vi "User Event.vi"() -> ()   [LabVIEW 2018]
doc: "This VI is an exercise in the LabVIEW Advanced course."
panel:
  out "이벤트 카운트":i16
  in  "정지":bool
  out "이벤트 발생!":bool
  in  "이벤트 발생":bool
  out "루프 1 정지":bool
  out "이벤트를 발생시키기 위한 프로그램적인 카운트 다운":u8(slide) scale=0.0..100.0
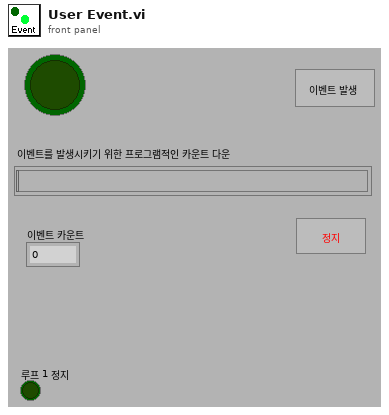
[diagram p1: front panel]
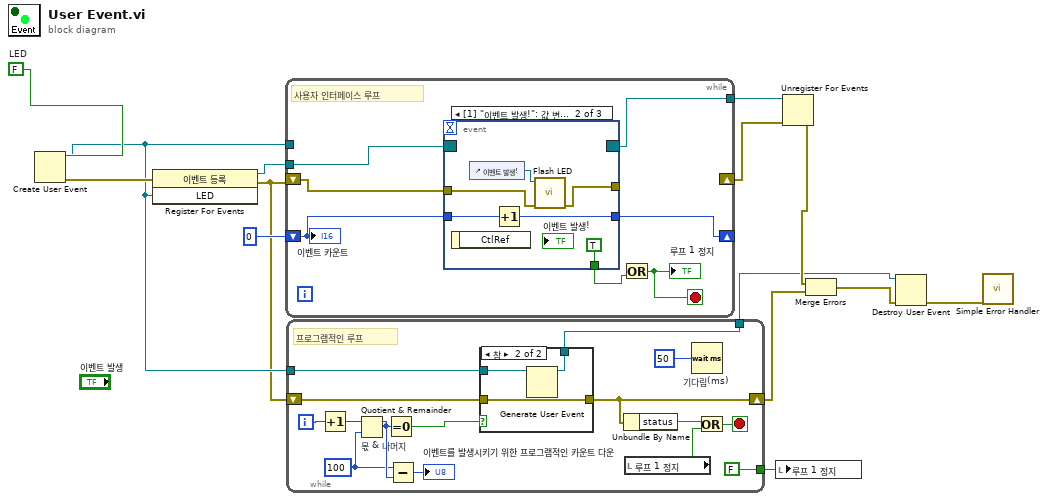
[diagram p0: block diagram]
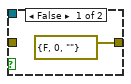
[diagram p2: hidden frame]
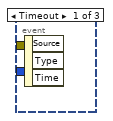
[diagram p3: hidden frame]
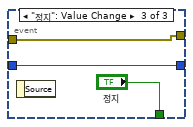
[diagram p4: hidden frame]
diagram:
  w12 = FALSE  # LED
  n1 = Create User Event(user event datatype=w12) -> (user event=w10:refnum<user-event>, error out=w11:errorcluster)  [unwired: 1 in]
  n2 = register-events(error in=w11, w10) -> (reference out=w8:refnum<event-registration>, error out=w9:errorcluster)  [unwired: 1 in]
  n3 = while {
    shift-right: [w18] -> _
    shift-left: i16 0 ("Event Count") -> [w19]
    tunnel: w10 -> [_]
    shift-right: [_] -> w7
    shift-left: w9 -> [w17]
    tunnel: w8 -> [w20]
    tunnel: [w15] -> w6
    stop <- w21 stop-if-true
    # "사용자 인터페이스 루프"
    n4 = event shown="[1] \"이벤트 발생!\": 값 변경" {
      selector: w20 -> [_ _ _]
      dyn-events: [_ _ _] -> w15
      timeout: _ -> [_ _ _]
      tunnel: w19 -> [_ w26 w29]
      tunnel: [_ w25 w29] -> w18
      tunnel: w17 -> [_ w24 w30]
      tunnel: [_ TRUE "정지"] -> w16
      tunnel: [_ w22 w30] -> _
      event Timeout {
        n5 = event-data() -> ()  [unwired: 1 in, 3 out]
      }
      event "이벤트 발생!": Value Change {
        n6 = event-data() -> ()  [unwired: 1 in, 1 out]
        n7 = control-ref of="이벤트 발생!"() -> (w27:refnum<vi>)
        n8 = Increment(x=w26) -> (x+1=w25:i16)
        n9 = call "Flash LED.vi"("에러 입력(에러 없음)"=w24, "Bool 참조번호"=w27) -> ("에러 출력"=w22:errorcluster)  [unwired: 5 in]
      }
      event "정지": Value Change {
        n10 = event-data() -> ()  [unwired: 1 in, 1 out]
      }
    }
    n11 = Or(y=w16) -> (x .or. y?=w21:bool)  [unwired: 1 in]
    "루프 1 정지" <- w21
    "이벤트 카운트" <- w19
  }
  n12 = while {
    shift-right: [w41] -> w3
    shift-left: w9 -> [w42]
    tunnel: [FALSE] -> w13
    tunnel: w10 -> [w32]
    tunnel: [w31] -> w1
    i -> [w44]
    stop <- w39 stop-if-true
    w33 = 100 ("y")
    # "프로그램적인 루프"
    n13 = Increment ("증가")(x=w44) -> (x+1=w35:i32)
    n14 = Quotient & Remainder "몫 & 나머지"(x=w35, y=w33) -> (x-y*floor(x/y)=w34:i32)  [unwired: 1 out]
    n15 = Equal To 0? ("0과 같음?")(x=w34) -> (x = 0?=w43:bool)
    n16 = Subtract ("빼기")(x=w33, y=w34) -> (x-y=→"이벤트를 발생시키기 위한 프로그램적인 카운트 다운":i32)
    n17 = case shown="참" w43 {
      tunnel: [errorcluster {"status"=FALSE, "code"=0, "source"=""} ("error out") w49] -> w41
      tunnel: w42 -> [_ w49]
      tunnel: w32 -> [_ w48]
      tunnel: [_ w47] -> w31
      frame False {
      }
      frame True {
        n18 = Generate User Event(user event=w48) -> (user event out=w47:refnum<user-event>)  [unwired: 3 in, 1 out]
      }
    }
    n19 = Unbundle By Name(w41) -> ("status"=w38:bool)
    n20 = local read "루프 1 정지"() -> (w37:bool)
    n21 = Wait (ms) "기다림(ms)"(milliseconds to wait=u32 50) -> ()  [unwired: 1 out]
    n22 = Or(x=w38, y=w37) -> (x .or. y?=w39:bool)
  }
  n23 = local write "루프 1 정지"(w13) -> ()
  n24 = Unregister For Events(event registration refnum=w6, error in=w7) -> (error out=w4:errorcluster)
  n25 = Merge Errors(w4, w3) -> (w2:errorcluster)
  n26 = Destroy User Event(user event=w1, error in=w2) -> (error out=w5:errorcluster)
  n27 = call <vilib>:"Simple Error Handler.vi"("error in (no error)"=w5) -> ()  [unwired: 4 in, 5 out]
